vi "Test_3_3vdc.vi"(8 "error in (no error)":errorcluster, 11 "Use AP1 (y)":bool=TRUE) -> (0 "error out":errorcluster, 1 "3.3vdc reading":dbl, 2 "read buffer":string, 3 "Passed?":bool)   [LabVIEW 2024]
uses:
  <vilib>/Instr/_visa.llb/VISA Configure Serial Port (Instr).vi
panel:
  out "ADC reading":string
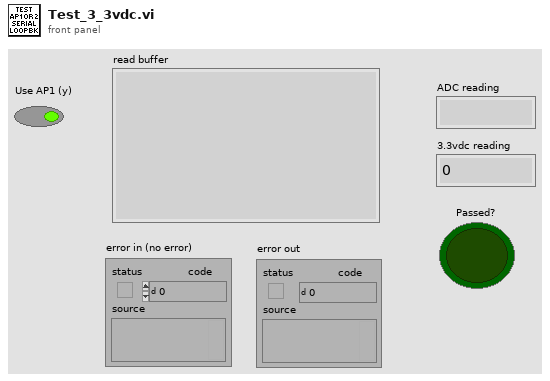
[diagram p1: front panel]
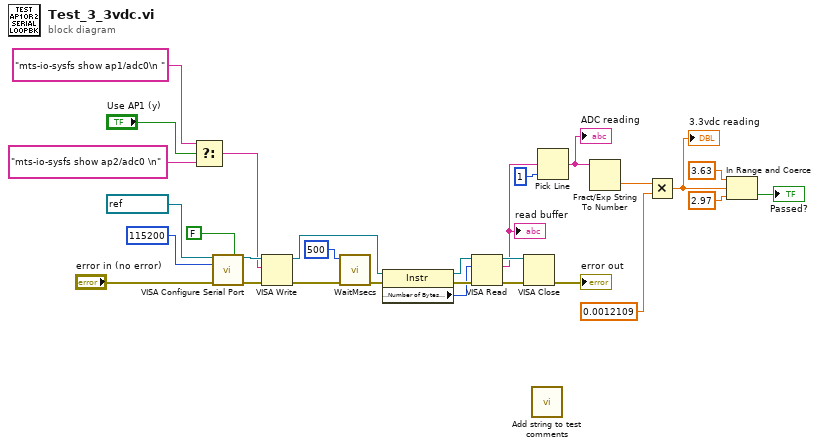
[diagram p0: block diagram]
diagram:
  n1 = Select(t="mts-io-sysfs show ap1/adc0\n ", s="Use AP1 (y)", f="mts-io-sysfs show ap2/adc0 \n") -> (s? t:f=w15:string)
  n2 = call-poly "VISA Configure Serial Port"("VISA resource name"=refnum<visa-resource-name> "COM5", "Enable Termination\nChar (T)"=FALSE ("Enable Termination\nChar (T)"), "baud rate (9600)"=u32 115200, "error in (no error)"="error in (no error)") -> ("VISA resource name out"=w25:refnum<visa-resource-name>, "error out"=w24:errorcluster)  [unwired: 10 in]
  n3 = VISA Write(VISA resource name=w25, write buffer=w15, error in (no error)=w24) -> (VISA resource name out=w12:refnum<visa-resource-name>, error out=w13:errorcluster)  [unwired: 1 out]
  n4 = call "WaitMsecs.vi"("error in (no error)"=w13, "Wait Msecs"=u32 500) -> ("error out"=w22:errorcluster)  [unwired: 9 in]
  n5 = property class="Instr"(reference=w12, error in=w22) -> (reference out=w21:refnum<visa-resource-name>, error out=w20:errorcluster, "Serial Settings:Number of Bytes at Serial Port"=w19:u32)
  n6 = VISA Read(VISA resource name=w21, byte count=w19, error in (no error)=w20) -> (VISA resource name out=w10:refnum<visa-resource-name>, read buffer=w9:string, error out=w11:errorcluster)  [unwired: 1 out]
  "read buffer" <- w9
  n7 = VISA Close(VISA resource name=w10, error in (no error)=w11) -> (error out=→"error out":errorcluster)
  n8 = call "Add string to test comments.vi"() -> ()  [unwired: 10 in, 2 out]
  n9 = Pick Line(multi-line string=w9, line index=1) -> (output string=w7:string)  [unwired: 1 in]
  "ADC reading" <- w7
  n10 = Fract/Exp String To Number(string=w7) -> (number=w6:dbl)  [unwired: 3 in, 1 out]
  n11 = Multiply(x=w6, y=0.0012109) -> (x*y=w4:dbl)
  "3.3vdc reading" <- w4
  n12 = In Range and Coerce(upper limit=3.63, x=w4, lower limit=2.97) -> (In Range?=→"Passed?":bool)  [unwired: 1 out]
